vi "old APU and old Event Timing v6 single shot.vi"() -> ()   [LabVIEW 2015]
uses:
  <vilib>/Platform/TimedLoop/XDataNode/wakeup.ctl
  <vilib>/Platform/TimedLoop/XDataNode/XDNodeRunTimeDep.lvlib
  <vilib>/Platform/TimedLoop/XDataNode/nitl_modes.ctl
  <vilib>/Platform/TimedLoop/XDataNode/timing_clust.ctl
  <vilib>/Platform/TimedLoop/XDataNode/XDataNode.xnode
  <userlib>/_NI VeriStand FPGA Support/NI VeriStand RIO Library/Custom Device Components/Engine Simulation/Engine Simulation Globals.vi
  <userlib>/AES/FPGA/FPGA VIs/AES ECU Event Measurement - All Measurements.vi
  <vilib>/eio/EIONode/EIONode.xnode
  <vilib>/rvi/eio/common/nirviEmuTemplateMethod_errors.vi
panel:
  out "ECUEvent.IC 1.End Angle":u64
  out "ECUEvent.IC 2.End Angle":u64
  out "ECUEvent.IC 3.End Angle":u64
  out "ECUEvent.IC 4.End Angle":u64
  out "ECUEvent.IC 5.End Angle":u64
  out "ECUEvent.IC 6.End Angle":u64
  out "ECUEvent.IC 1.Time Duration":u32
  out "ECUEvent.IC 1.Start Angle":u64
  out "ECUEvent.IC 1.Angle Duration":u64
  out "ECUEvent.IC 2.Time Duration":u32
  out "ECUEvent.IC 2.Start Angle":u64
  out "ECUEvent.IC 2.Angle Duration":u64
  out "ECUEvent.IC 3.Time Duration":u32
  out "ECUEvent.IC 3.Start Angle":u64
  out "ECUEvent.IC 3.Angle Duration":u64
  out "ECUEvent.IC 4.Time Duration":u32
  out "ECUEvent.IC 4.Start Angle":u64
  out "ECUEvent.IC 4.Angle Duration":u64
  out "ECUEvent.IC 5.Time Duration":u32
  out "ECUEvent.IC 5.Start Angle":u64
  out "ECUEvent.IC 5.Angle Duration":u64
  out "ECUEvent.IC 6.Time Duration":u32
  out "ECUEvent.IC 6.Start Angle":u64
  out "ECUEvent.IC 6.Angle Duration":u64
  out "ECUEvent.FI 1.End Angle":u64
  out "ECUEvent.FI 2.End Angle":u64
  out "ECUEvent.FI 3.End Angle":u64
  out "ECUEvent.FI 4.End Angle":u64
  out "ECUEvent.FI 5.End Angle":u64
  out "ECUEvent.FI 6.End Angle":u64
  out "ECUEvent.FI 1.Time Duration":u32
  out "ECUEvent.FI 1.Start Angle":u64
  out "ECUEvent.FI 1.Angle Duration":u64
  out "ECUEvent.FI 2.Time Duration":u32
  out "ECUEvent.FI 2.Start Angle":u64
  out "ECUEvent.FI 2.Angle Duration":u64
  out "ECUEvent.FI 3.Time Duration":u32
  out "ECUEvent.FI 3.Start Angle":u64
  out "ECUEvent.FI 3.Angle Duration":u64
  out "ECUEvent.FI 4.Time Duration":u32
  out "ECUEvent.FI 4.Start Angle":u64
  out "ECUEvent.FI 4.Angle Duration":u64
  out "ECUEvent.FI 5.Time Duration":u32
  out "ECUEvent.FI 5.Start Angle":u64
  out "ECUEvent.FI 5.Angle Duration":u64
  out "ECUEvent.FI 6.Time Duration":u32
  out "ECUEvent.FI 6.Start Angle":u64
  out "ECUEvent.FI 6.Angle Duration":u64
  in  "APU.Degrees per Tick":u64
  out "APU.Crank Angle":u64
  out "APU.Cycle Angle":u64
  in  "APU.Reset":bool
  in  "APU.Increment Rate":u64
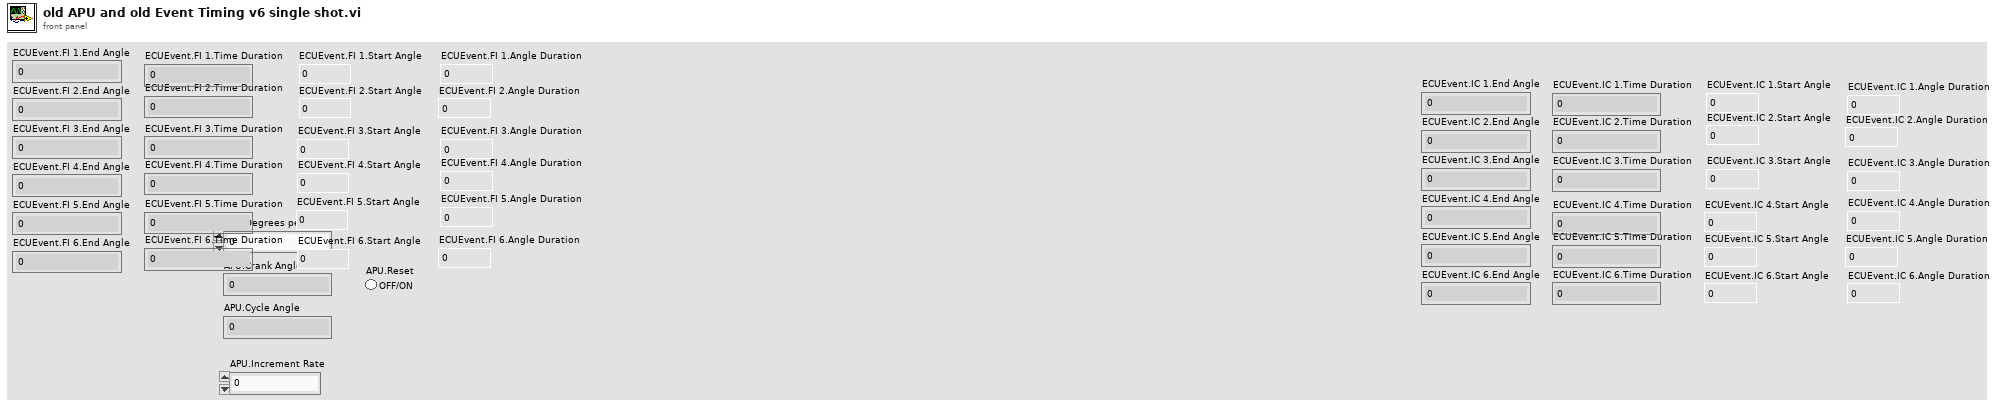
[diagram p1: front panel]
types:
  T1 = typedef "XDNodeRunTimeDep.lvlib/timing_clust.ctl" = cluster{"Expected End [f-1]":u64, "Actual End [f-1]":u64, "Finished Late? [f-1]":bool, "Expected End [i-1]":u64, "Actual End [i-1]":u64, "Finished Late? [i-1]":bool, "Expected Start [i]":u64, "Actual Start [i]":u64, "Expected Start [f]":u64, "Actual Start [f]":u64, "Source Name":string, "Structure Name":string, "Period":i64, "Deadline":i64, "Offset":i64, "Start":i64, "Priority":i32, "Timeout":i32, "Mode":T2, "Wakeup Reason":T3, "Error":errorcluster, "Source Type":string, "Secondary Source Type":string, "Global End Time":u64, "Global Start Time":u64, "Frame Duration":u64, "Iteration Duration":u64, "Assigned CPU":i32, "I/O Scan Engine Mode":u32}
  T2 = typedef "XDNodeRunTimeDep.lvlib/nitl_modes.ctl" = enum32{"No Change", "Process missed periods, maintain original phase", "Discard missed periods, maintain original phase", "Process missed periods, ignore original phase", "Discard missed periods, ignore original phase"}
  T3 = typedef "XDNodeRunTimeDep.lvlib/wakeup.ctl" = enum32{"Normal", "Aborted", "Asynchronous wakeup", "Timing source error", "Timed loop error", "Timeout"}
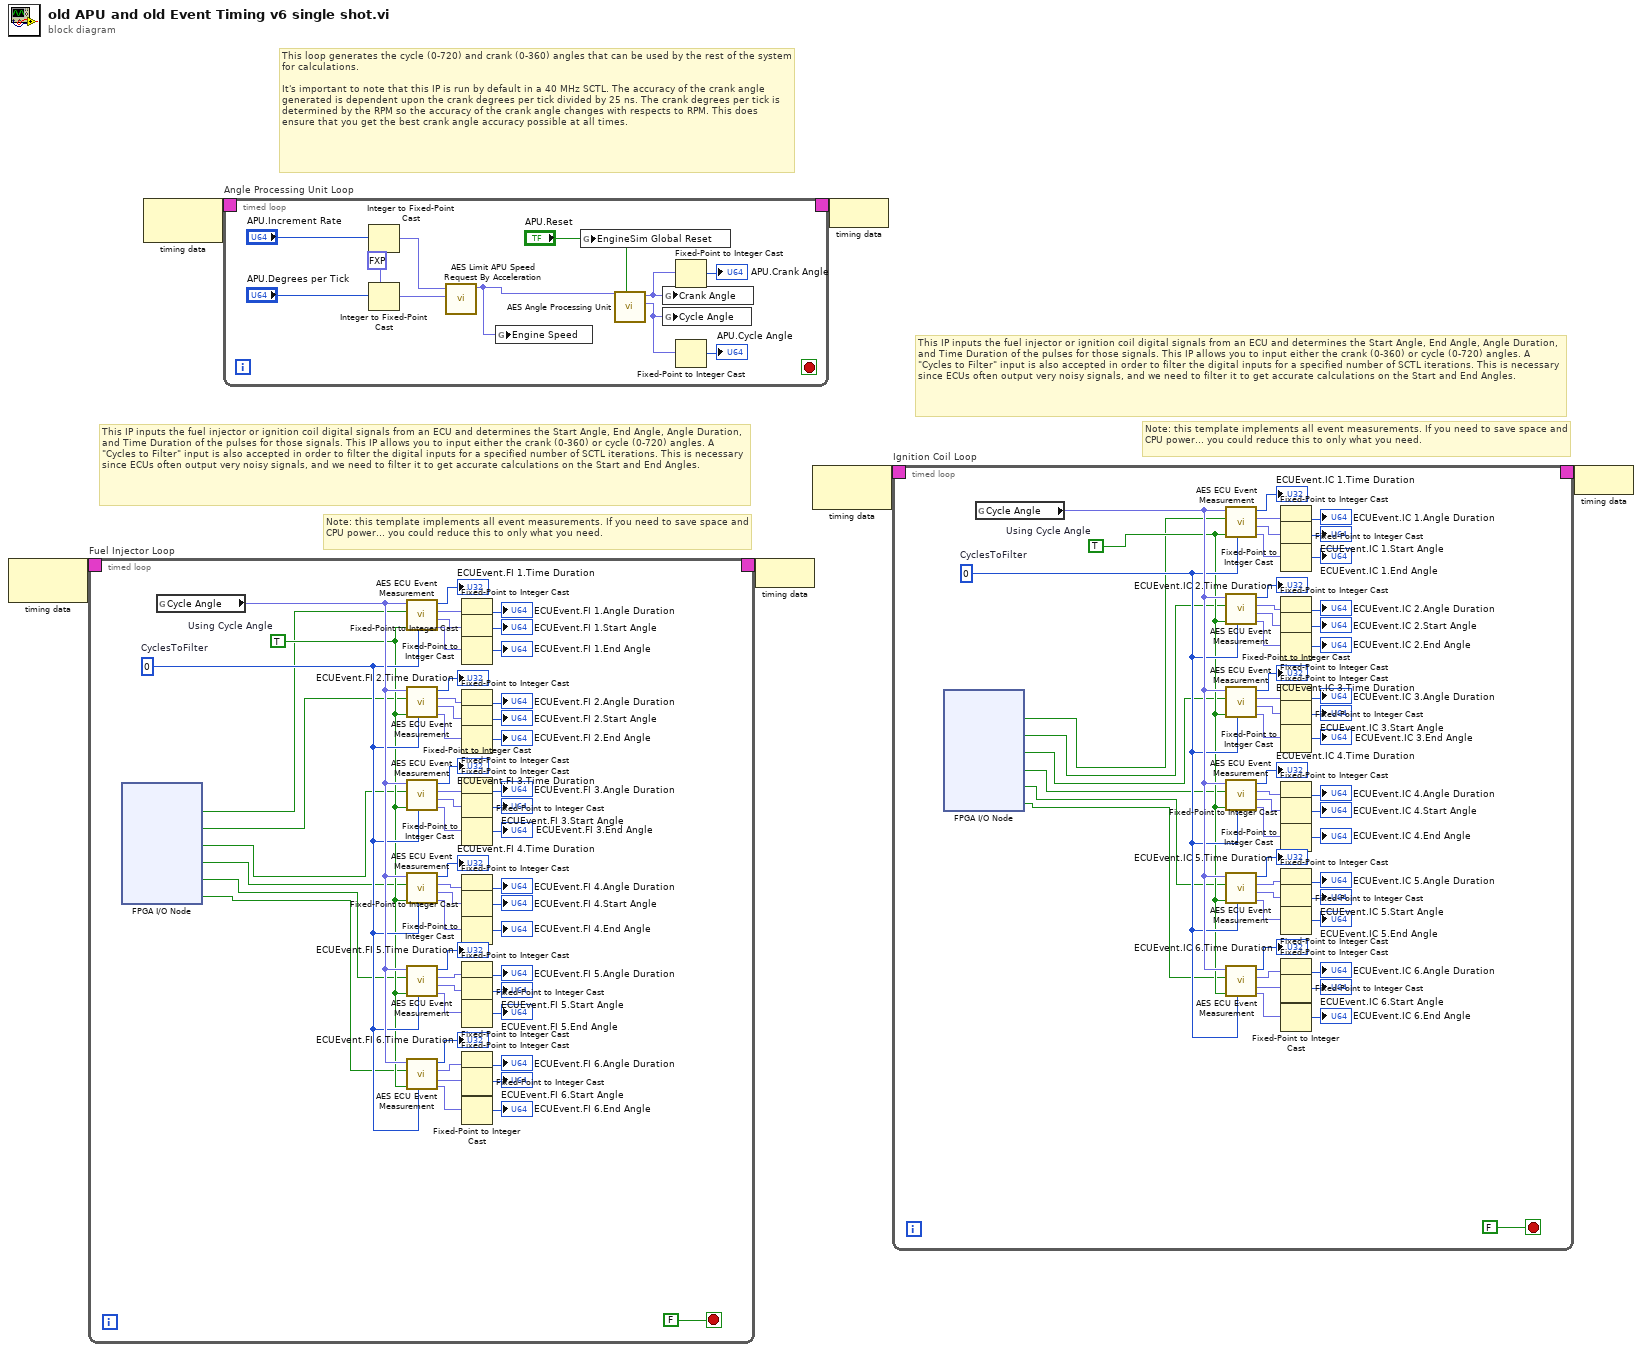
[diagram p0: block diagram]
diagram:
  # "Note: this template implements all event measurements. If you need to save space and CPU power... you could reduce this to only what you need."
  # "This IP inputs the fuel injector or ignition coil digital signals from an ECU and determines the Start Angle, End Angle, Angle Duration, and Time Duration of the pulses for those signals. This IP allows you to input either the crank (0-360) or cycle (0-720) angles. A \"Cycles to Filter\" input is also accepted in order to filter the digital inputs for a specified number of SCTL iterations. This is necessary since ECUs often output very noisy signals, and we need to filter it to get accurate calculations on the Start and End Angles."
  # "Note: this template implements all event measurements. If you need to save space and CPU power... you could reduce this to only what you need."
  # "This IP inputs the fuel injector or ignition coil digital signals from an ECU and determines the Start Angle, End Angle, Angle Duration, and Time Duration of the pulses for those signals. This IP allows you to input either the crank (0-360) or cycle (0-720) angles. A \"Cycles to Filter\" input is also accepted in order to filter the digital inputs for a specified number of SCTL iterations. This is necessary since ECUs often output very noisy signals, and we need to filter it to get accurate calculations on the Start and End Angles."
  # "This loop generates the cycle (0-720) and crank (0-360) angles that can be used by the rest of the system for calculations. \n\nIt's important to note that this IP is run by default in a 40 MHz SCTL. The accuracy of the crank angle generated is dependent upon the crank degrees per tick divided by 25 ns. The crank degrees per tick is determined by the RPM so the accuracy of the crank angle changes with respects to RPM. This does ensure that you get the best crank angle accuracy possible at all times."
  n1 = node-c288() -> (w4:T1)  [unwired: 1 out]
  n2 = timed-loop "Fuel Injector Loop" {
    timing: w4 -> [_]
    timing-out: [_] -> w3
    stop <- FALSE stop-if-true
    w13 = TRUE  # Using Cycle Angle
    w56 = u16 0  # CyclesToFilter
    n3 = xnode "FPGA I/O Node"() -> ("DIO0_0"=w12:bool, "DIO1_0"=w11:bool, "DIO2_0"=w10:bool, "DIO3_0"=w9:bool, "DIO4_0"=w8:bool, "DIO5_0"=w7:bool)  [unwired: 6 in, 6 out]
    n4 = global read "Engine Simulation Globals.vi" "Cycle Angle"() -> (w57:fxp<+,61,10>)
    n5 = call-poly <userlib>:"AES ECU Event Measurement.vi"("Cycles to Filter"=w56, "Using Cycle Angle"=w13, "Digital Input Pulse"=w12, "Crank or Cyle Angle"=w57) -> ("End Angle (degrees)"=w49:fxp<+,61,10>, "Start Angle (degrees)"=w44:fxp<+,61,10>, "Angle Duration (degrees)"=w43:fxp<+/-,62,11>, "Time Duration (clock ticks)"=→"ECUEvent.FI 1.Time Duration":u32)  [unwired: 4 in]
    n6 = call-poly <userlib>:"AES ECU Event Measurement.vi"("Cycles to Filter"=w56, "Using Cycle Angle"=w13, "Digital Input Pulse"=w11, "Crank or Cyle Angle"=w57) -> ("End Angle (degrees)"=w48:fxp<+,61,10>, "Start Angle (degrees)"=w38:fxp<+,61,10>, "Angle Duration (degrees)"=w37:fxp<+/-,62,11>, "Time Duration (clock ticks)"=→"ECUEvent.FI 2.Time Duration":u32)  [unwired: 4 in]
    n7 = call-poly <userlib>:"AES ECU Event Measurement.vi"("Cycles to Filter"=w56, "Using Cycle Angle"=w13, "Digital Input Pulse"=w10, "Crank or Cyle Angle"=w57) -> ("End Angle (degrees)"=w47:fxp<+,61,10>, "Start Angle (degrees)"=w32:fxp<+,61,10>, "Angle Duration (degrees)"=w31:fxp<+/-,62,11>, "Time Duration (clock ticks)"=→"ECUEvent.FI 3.Time Duration":u32)  [unwired: 4 in]
    n8 = call-poly <userlib>:"AES ECU Event Measurement.vi"("Cycles to Filter"=w56, "Using Cycle Angle"=w13, "Digital Input Pulse"=w9, "Crank or Cyle Angle"=w57) -> ("End Angle (degrees)"=w46:fxp<+,61,10>, "Start Angle (degrees)"=w25:fxp<+,61,10>, "Angle Duration (degrees)"=w26:fxp<+/-,62,11>, "Time Duration (clock ticks)"=→"ECUEvent.FI 4.Time Duration":u32)  [unwired: 4 in]
    n9 = call-poly <userlib>:"AES ECU Event Measurement.vi"("Cycles to Filter"=w56, "Using Cycle Angle"=w13, "Digital Input Pulse"=w8, "Crank or Cyle Angle"=w57) -> ("End Angle (degrees)"=w45:fxp<+,61,10>, "Start Angle (degrees)"=w22:fxp<+,61,10>, "Angle Duration (degrees)"=w21:fxp<+/-,62,11>, "Time Duration (clock ticks)"=→"ECUEvent.FI 5.Time Duration":u32)  [unwired: 4 in]
    n10 = call-poly <userlib>:"AES ECU Event Measurement.vi"("Cycles to Filter"=w56, "Using Cycle Angle"=w13, "Digital Input Pulse"=w7, "Crank or Cyle Angle"=w57) -> ("End Angle (degrees)"=w18:fxp<+,61,10>, "Start Angle (degrees)"=w16:fxp<+,61,10>, "Angle Duration (degrees)"=w17:fxp<+/-,62,11>, "Time Duration (clock ticks)"=→"ECUEvent.FI 6.Time Duration":u32)  [unwired: 4 in]
    n11 = Fixed-Point to Integer Cast(1:w43) -> (0:→"ECUEvent.FI 1.Angle Duration":i64)
    n12 = Fixed-Point to Integer Cast(1:w44) -> (0:→"ECUEvent.FI 1.Start Angle":u64)
    n13 = Fixed-Point to Integer Cast(1:w49) -> (0:→"ECUEvent.FI 1.End Angle":u64)
    n14 = Fixed-Point to Integer Cast(1:w37) -> (0:→"ECUEvent.FI 2.Angle Duration":i64)
    n15 = Fixed-Point to Integer Cast(1:w38) -> (0:→"ECUEvent.FI 2.Start Angle":u64)
    n16 = Fixed-Point to Integer Cast(1:w48) -> (0:→"ECUEvent.FI 2.End Angle":u64)
    n17 = Fixed-Point to Integer Cast(1:w31) -> (0:→"ECUEvent.FI 3.Angle Duration":i64)
    n18 = Fixed-Point to Integer Cast(1:w32) -> (0:→"ECUEvent.FI 3.Start Angle":u64)
    n19 = Fixed-Point to Integer Cast(1:w47) -> (0:→"ECUEvent.FI 3.End Angle":u64)
    n20 = Fixed-Point to Integer Cast(1:w26) -> (0:→"ECUEvent.FI 4.Angle Duration":i64)
    n21 = Fixed-Point to Integer Cast(1:w25) -> (0:→"ECUEvent.FI 4.Start Angle":u64)
    n22 = Fixed-Point to Integer Cast(1:w46) -> (0:→"ECUEvent.FI 4.End Angle":u64)
    n23 = Fixed-Point to Integer Cast(1:w21) -> (0:→"ECUEvent.FI 5.Angle Duration":i64)
    n24 = Fixed-Point to Integer Cast(1:w22) -> (0:→"ECUEvent.FI 5.Start Angle":u64)
    n25 = Fixed-Point to Integer Cast(1:w45) -> (0:→"ECUEvent.FI 5.End Angle":u64)
    n26 = Fixed-Point to Integer Cast(1:w17) -> (0:→"ECUEvent.FI 6.Angle Duration":i64)
    n27 = Fixed-Point to Integer Cast(1:w16) -> (0:→"ECUEvent.FI 6.Start Angle":u64)
    n28 = Fixed-Point to Integer Cast(1:w18) -> (0:→"ECUEvent.FI 6.End Angle":u64)
  }
  n29 = node-c288() -> (w6:T1)  [unwired: 1 in]
  n30 = timed-loop "Angle Processing Unit Loop" {
    timing: w6 -> [_]
    timing-out: [_] -> w5
    stop <- _ stop-if-true
    w63 = fxp<+/-,47,-4> 0.0 ("Crank.Degrees per Tick")
    n31 = Integer to Fixed-Point Cast(fixed-point type=w63, integer="APU.Increment Rate") -> (fixed-point=w62:fxp<+/-,47,-4>)
    n32 = Integer to Fixed-Point Cast(fixed-point type=w63, integer="APU.Degrees per Tick") -> (fixed-point=w65:fxp<+/-,47,-4>)
    n33 = call <userlib>:"AES Limit APU Speed Request By Acceleration.vi"("APU.Degrees per Tick in"=w65, "APU.Increment Rate"=w62) -> ("APU.Degrees per Tick out"=w61:fxp<+/-,47,-4>)  [unwired: 9 in]
    n34 = global write "Engine Simulation Globals.vi" "Engine Speed"(w61) -> ()
    n35 = global write "Engine Simulation Globals.vi" "EngineSim Global Reset"("APU.Reset") -> ()
    n36 = call <userlib>:"AES Angle Processing Unit.vi"("APU.Reset"="APU.Reset", "APU.Degrees per Tick"=w61) -> ("APU.Cycle Angle"=w67:fxp<+,61,10>, "APU.Crank Angle"=w71:fxp<+,60,9>)  [unwired: 8 in]
    n37 = global write "Engine Simulation Globals.vi" "Crank Angle"(w71) -> ()
    n38 = global write "Engine Simulation Globals.vi" "Cycle Angle"(w67) -> ()
    n39 = Fixed-Point to Integer Cast(1:w71) -> (0:→"APU.Crank Angle":u64)
    n40 = Fixed-Point to Integer Cast(1:w67) -> (0:→"APU.Cycle Angle":u64)
  }
  n41 = node-c288(w3) -> ()
  n42 = node-c288() -> (w2:T1)  [unwired: 1 out]
  n43 = node-c288(w5) -> ()
  n44 = timed-loop "Ignition Coil Loop" {
    timing: w2 -> [_]
    timing-out: [_] -> w1
    stop <- FALSE stop-if-true
    w80 = TRUE  # Using Cycle Angle
    w123 = u16 0  # CyclesToFilter
    n45 = xnode "FPGA I/O Node"() -> ("DIO0_1"=w79:bool, "DIO1_1"=w78:bool, "DIO2_1"=w77:bool, "DIO3_1"=w76:bool, "DIO4_1"=w75:bool, "DIO5_1"=w74:bool)  [unwired: 6 in, 6 out]
    n46 = global read "Engine Simulation Globals.vi" "Cycle Angle"() -> (w124:fxp<+,61,10>)
    n47 = call-poly <userlib>:"AES ECU Event Measurement.vi"("Cycles to Filter"=w123, "Using Cycle Angle"=w80, "Digital Input Pulse"=w79, "Crank or Cyle Angle"=w124) -> ("End Angle (degrees)"=w116:fxp<+,61,10>, "Start Angle (degrees)"=w111:fxp<+,61,10>, "Angle Duration (degrees)"=w110:fxp<+/-,62,11>, "Time Duration (clock ticks)"=→"ECUEvent.IC 1.Time Duration":u32)  [unwired: 4 in]
    n48 = call-poly <userlib>:"AES ECU Event Measurement.vi"("Cycles to Filter"=w123, "Using Cycle Angle"=w80, "Digital Input Pulse"=w78, "Crank or Cyle Angle"=w124) -> ("End Angle (degrees)"=w115:fxp<+,61,10>, "Start Angle (degrees)"=w105:fxp<+,61,10>, "Angle Duration (degrees)"=w104:fxp<+/-,62,11>, "Time Duration (clock ticks)"=→"ECUEvent.IC 2.Time Duration":u32)  [unwired: 4 in]
    n49 = call-poly <userlib>:"AES ECU Event Measurement.vi"("Cycles to Filter"=w123, "Using Cycle Angle"=w80, "Digital Input Pulse"=w77, "Crank or Cyle Angle"=w124) -> ("End Angle (degrees)"=w114:fxp<+,61,10>, "Start Angle (degrees)"=w99:fxp<+,61,10>, "Angle Duration (degrees)"=w98:fxp<+/-,62,11>, "Time Duration (clock ticks)"=→"ECUEvent.IC 3.Time Duration":u32)  [unwired: 4 in]
    n50 = call-poly <userlib>:"AES ECU Event Measurement.vi"("Cycles to Filter"=w123, "Using Cycle Angle"=w80, "Digital Input Pulse"=w76, "Crank or Cyle Angle"=w124) -> ("End Angle (degrees)"=w113:fxp<+,61,10>, "Start Angle (degrees)"=w92:fxp<+,61,10>, "Angle Duration (degrees)"=w93:fxp<+/-,62,11>, "Time Duration (clock ticks)"=→"ECUEvent.IC 4.Time Duration":u32)  [unwired: 4 in]
    n51 = call-poly <userlib>:"AES ECU Event Measurement.vi"("Cycles to Filter"=w123, "Using Cycle Angle"=w80, "Digital Input Pulse"=w75, "Crank or Cyle Angle"=w124) -> ("End Angle (degrees)"=w112:fxp<+,61,10>, "Start Angle (degrees)"=w89:fxp<+,61,10>, "Angle Duration (degrees)"=w88:fxp<+/-,62,11>, "Time Duration (clock ticks)"=→"ECUEvent.IC 5.Time Duration":u32)  [unwired: 4 in]
    n52 = call-poly <userlib>:"AES ECU Event Measurement.vi"("Cycles to Filter"=w123, "Using Cycle Angle"=w80, "Digital Input Pulse"=w74, "Crank or Cyle Angle"=w124) -> ("End Angle (degrees)"=w85:fxp<+,61,10>, "Start Angle (degrees)"=w83:fxp<+,61,10>, "Angle Duration (degrees)"=w84:fxp<+/-,62,11>, "Time Duration (clock ticks)"=→"ECUEvent.IC 6.Time Duration":u32)  [unwired: 4 in]
    n53 = Fixed-Point to Integer Cast(1:w110) -> (0:→"ECUEvent.IC 1.Angle Duration":i64)
    n54 = Fixed-Point to Integer Cast(1:w111) -> (0:→"ECUEvent.IC 1.Start Angle":u64)
    n55 = Fixed-Point to Integer Cast(1:w116) -> (0:→"ECUEvent.IC 1.End Angle":u64)
    n56 = Fixed-Point to Integer Cast(1:w104) -> (0:→"ECUEvent.IC 2.Angle Duration":i64)
    n57 = Fixed-Point to Integer Cast(1:w105) -> (0:→"ECUEvent.IC 2.Start Angle":u64)
    n58 = Fixed-Point to Integer Cast(1:w115) -> (0:→"ECUEvent.IC 2.End Angle":u64)
    n59 = Fixed-Point to Integer Cast(1:w98) -> (0:→"ECUEvent.IC 3.Angle Duration":i64)
    n60 = Fixed-Point to Integer Cast(1:w99) -> (0:→"ECUEvent.IC 3.Start Angle":u64)
    n61 = Fixed-Point to Integer Cast(1:w114) -> (0:→"ECUEvent.IC 3.End Angle":u64)
    n62 = Fixed-Point to Integer Cast(1:w93) -> (0:→"ECUEvent.IC 4.Angle Duration":i64)
    n63 = Fixed-Point to Integer Cast(1:w92) -> (0:→"ECUEvent.IC 4.Start Angle":u64)
    n64 = Fixed-Point to Integer Cast(1:w113) -> (0:→"ECUEvent.IC 4.End Angle":u64)
    n65 = Fixed-Point to Integer Cast(1:w88) -> (0:→"ECUEvent.IC 5.Angle Duration":i64)
    n66 = Fixed-Point to Integer Cast(1:w89) -> (0:→"ECUEvent.IC 5.Start Angle":u64)
    n67 = Fixed-Point to Integer Cast(1:w112) -> (0:→"ECUEvent.IC 5.End Angle":u64)
    n68 = Fixed-Point to Integer Cast(1:w84) -> (0:→"ECUEvent.IC 6.Angle Duration":i64)
    n69 = Fixed-Point to Integer Cast(1:w83) -> (0:→"ECUEvent.IC 6.Start Angle":u64)
    n70 = Fixed-Point to Integer Cast(1:w85) -> (0:→"ECUEvent.IC 6.End Angle":u64)
  }
  n71 = node-c288(w1) -> ()
